vi "Get BasePath.vi"(8 "error in (no error)":errorcluster, 11 "ErrorHandler in":refnum<class "ErrorHandler.lvclass">) -> (0 "error out":errorcluster, 2 "ErrorLogBasePath":path, 3 "ErrorHandler out":refnum<class "ErrorHandler.lvclass">)   [LabVIEW 2017, in "ErrorHandler.lvclass"]
doc: "Developed by Kevin Thompson\nkevin@thompsonengineering.net\n\nCopyright 2018\nThompson Engineering, LLC"
uses:
  ErrorHandler.lvclass
  ErrorHandler.lvclass/ErrorHandler.ctl
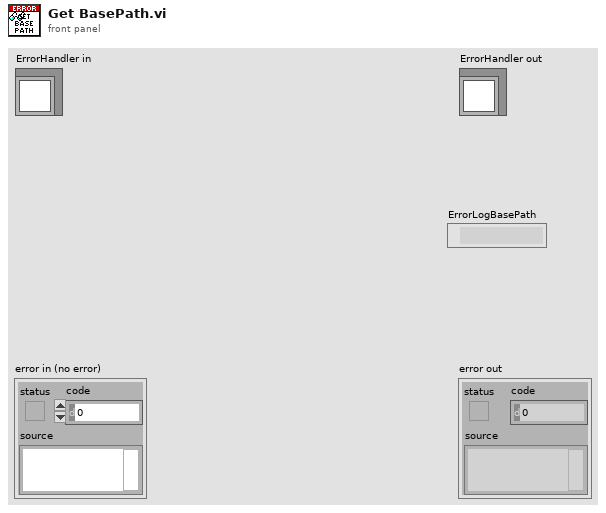
[diagram p1: front panel]
types:
  T1 = typedef "ErrorHandler.lvclass/ObjData--cluster.ctl" = cluster{"AppName":string, "ErrorLogBasePath":path, "ErrorDialogPopUp Disabled":bool, "TerminateAppOnError Enabled":bool}
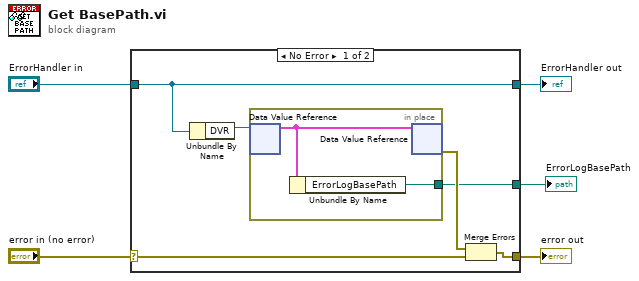
[diagram p0: block diagram]
diagram:
  n1 = case shown="No Error" "error in (no error)" {
    selector: "error in (no error)" -> [w11 w14]
    tunnel: [w8 w14] -> w4
    tunnel: [w10 w15] -> w2
    tunnel: "ErrorHandler in" -> [w10 w15]
    tunnel: [w6 _] -> w1
    frame No Error {
      n2 = Unbundle By Name(w10) -> ("DVR"=w9:refnum<data-value>)
      n3 = in-place {
        in-place-border: [w12] -> w6
        n4 = in-place-dvr #1(w9) -> (w13:T1)  [unwired: 1 out]
        n5 = Unbundle By Name(w13) -> ("ErrorLogBasePath"=w12:path)
        n6 = in-place-dvr #1(w13) -> (w7:errorcluster)  [unwired: 1 out]
      }
      n7 = Merge Errors(w7, w11) -> (w8:errorcluster)
    }
    frame Error {
    }
  }
  "error out" <- w4
  "ErrorHandler out" <- w2
  "ErrorLogBasePath" <- w1
